vi "calc.vi"() -> ()   [LabVIEW 2021]
panel:
  out "!result!":string
  in  "Enum":T1(ring)
  out "bin_num2":string
  out "bin_num1":string
  in  "!count!":bool
  out "operation type":string
  out "String":string
  in  "num2":dbl
  in  "num1":dbl
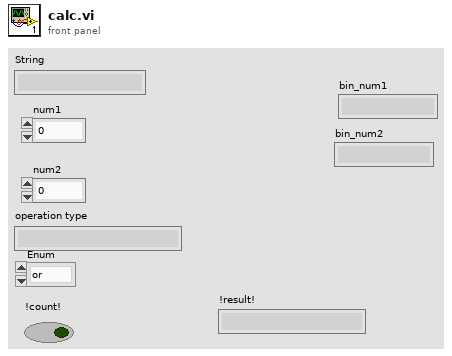
[diagram p1: front panel]
types:
  T1 = enum16{"or", "and", "not-or", "not-and", "exclusive or", "+", "-", "*"}
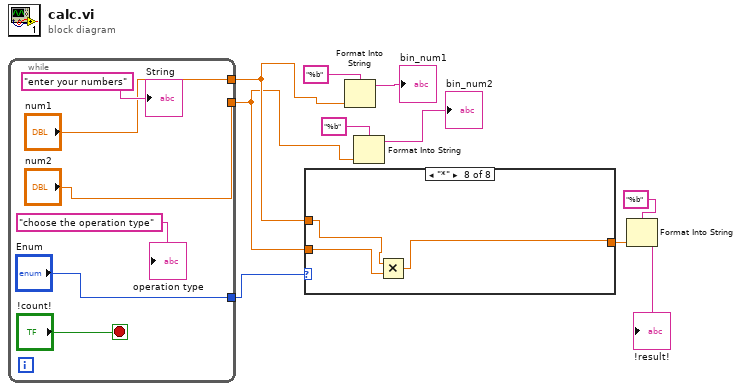
[diagram p0: block diagram]
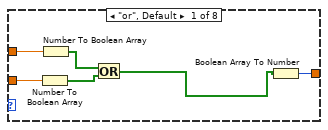
[diagram p2: hidden frame]
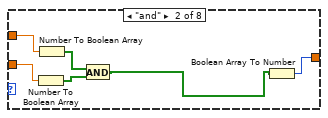
[diagram p3: hidden frame]
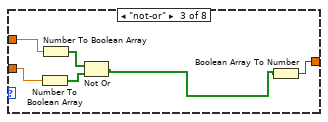
[diagram p4: hidden frame]
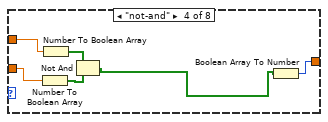
[diagram p5: hidden frame]
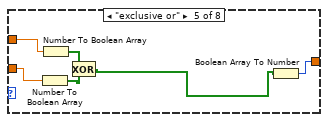
[diagram p6: hidden frame]
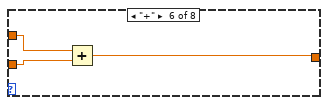
[diagram p7: hidden frame]
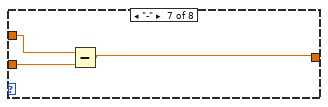
[diagram p8: hidden frame]
diagram:
  n1 = while {
    tunnel: ["num1"] -> w5
    tunnel: ["num2"] -> w4
    tunnel: ["Enum"] -> w6
    stop <- "!count!" stop-if-true
    "String" <- "enter your numbers" ("String")
    "operation type" <- "choose the operation type" ("String")
  }
  n2 = case shown="\"*\"" w6 {
    tunnel: w5 -> [w22 w28 w34 w40 w46 w49 w52 w55]
    tunnel: w4 -> [w21 w27 w33 w39 w45 w48 w51 w54]
    tunnel: [w18 w23 w29 w38 w44 w47 w50 w53] -> w1
    frame "or", Default {
      n3 = Number To Boolean Array(number=w21) -> (Boolean array=w19:bool[])
      n4 = Number To Boolean Array(number=w22) -> (Boolean array=w20:bool[])
      n5 = Or(x=w20, y=w19) -> (x .or. y?=w17:bool[])
      n6 = Boolean Array To Number(Boolean array=w17) -> (number=w18:u32)
    }
    frame "and" {
      n7 = Number To Boolean Array(number=w27) -> (Boolean array=w24:bool[])
      n8 = Number To Boolean Array(number=w28) -> (Boolean array=w25:bool[])
      n9 = And(x=w25, y=w24) -> (x .and. y?=w26:bool[])
      n10 = Boolean Array To Number(Boolean array=w26) -> (number=w23:u32)
    }
    frame "not-or" {
      n11 = Number To Boolean Array(number=w33) -> (Boolean array=w30:bool[])
      n12 = Number To Boolean Array(number=w34) -> (Boolean array=w31:bool[])
      n13 = Not Or(1:w30, 2:w31) -> (0:w32:bool[])
      n14 = Boolean Array To Number(Boolean array=w32) -> (number=w29:u32)
    }
    frame "not-and" {
      n15 = Number To Boolean Array(number=w39) -> (Boolean array=w36:bool[])
      n16 = Number To Boolean Array(number=w40) -> (Boolean array=w37:bool[])
      n17 = Not And(1:w36, 2:w37) -> (0:w35:bool[])
      n18 = Boolean Array To Number(Boolean array=w35) -> (number=w38:u32)
    }
    frame "exclusive or" {
      n19 = Number To Boolean Array(number=w45) -> (Boolean array=w41:bool[])
      n20 = Number To Boolean Array(number=w46) -> (Boolean array=w42:bool[])
      n21 = Exclusive Or(1:w41, 2:w42) -> (0:w43:bool[])
      n22 = Boolean Array To Number(Boolean array=w43) -> (number=w44:u32)
    }
    frame "+" {
      n23 = Add(x=w49, y=w48) -> (x+y=w47:dbl)
    }
    frame "-" {
      n24 = Subtract(x=w52, y=w51) -> (x-y=w50:dbl)
    }
    frame "*" {
      n25 = Multiply(x=w55, y=w54) -> (x*y=w53:dbl)
    }
  }
  n26 = Format Into String(format string="%b", w5) -> (resulting string=→"bin_num1":string)  [unwired: 2 in, 1 out]
  n27 = Format Into String(format string="%b", w4) -> (resulting string=→"bin_num2":string)  [unwired: 2 in, 1 out]
  n28 = Format Into String(format string="%b", w1) -> (resulting string=→"!result!":string)  [unwired: 2 in, 1 out]
